vi "TLM.vi"(4 "Error In":errorcluster, 7 "Command":string) -> (0 "Error Out":errorcluster, 3 "Response":string)   [LabVIEW 2018]
uses:
  MOKO_LabViewLibrary/MokoLowLevel/MokoLowLovelControl/MLLC_Mode.ctl
  data/TLM.ctl
panel:
  in  "Utility name":string="TLM"
  in  "Error Code":i32=5475
  in  "Settings":T2
  in  "Mode":T3=enum."Check"
  # "TLM"
  # "Default Settings"
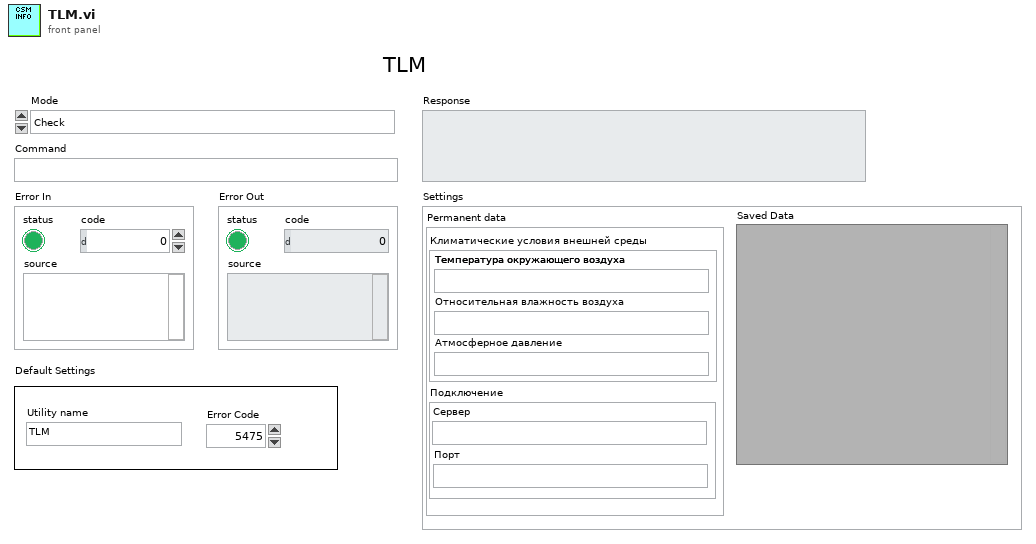
[diagram p1: front panel]
types:
  T1 = typedef "TLM.ctl" = cluster{"Климатические условия внешней среды":cluster{"Температура окружающего воздуха":string, "Относительная влажность воздуха":string, "Атмосферное давление":string}, "Подключение":cluster{"Сервер":string, "Порт":string}}
  T2 = cluster{"Saved Data":variant, "Permanent data":T1}
  T3 = typedef "MLLC_Mode.ctl" = enum16{"get", "set", "close", "Init", "Check"}
  T4 = typedef "MLLC_Error.ctl" = errorcluster
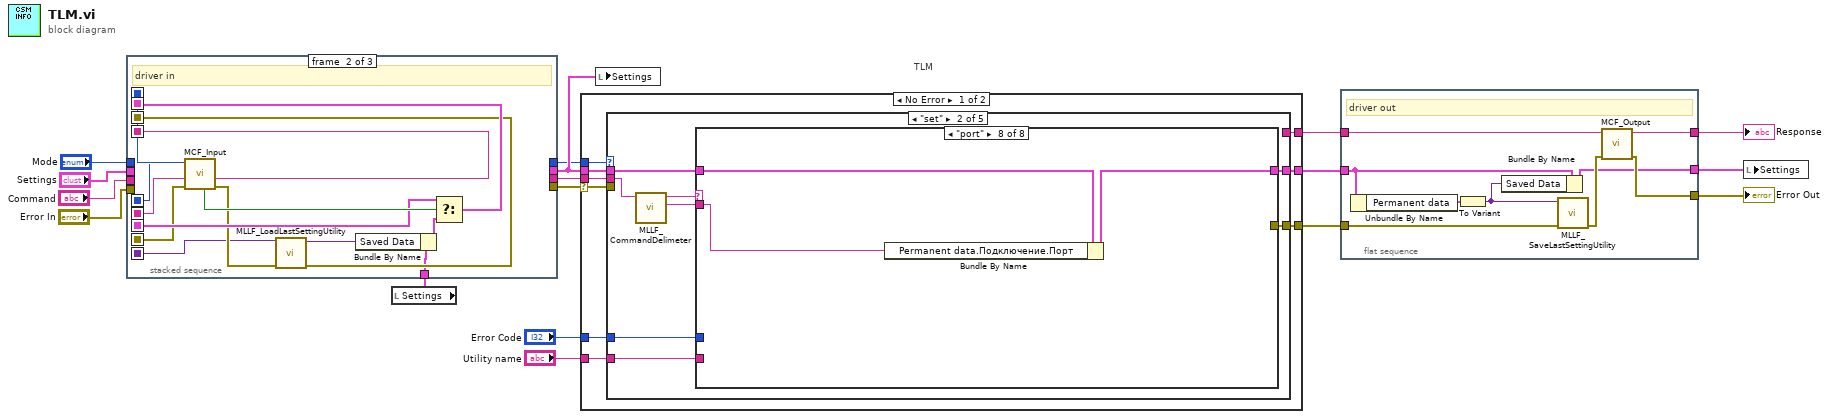
[diagram p0: block diagram]
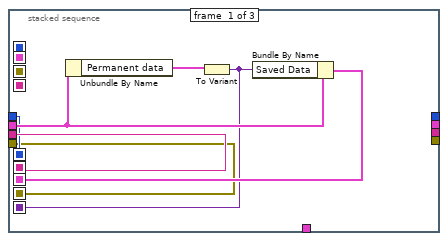
[diagram p2: hidden frame]
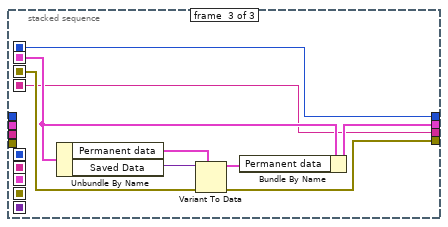
[diagram p3: hidden frame]
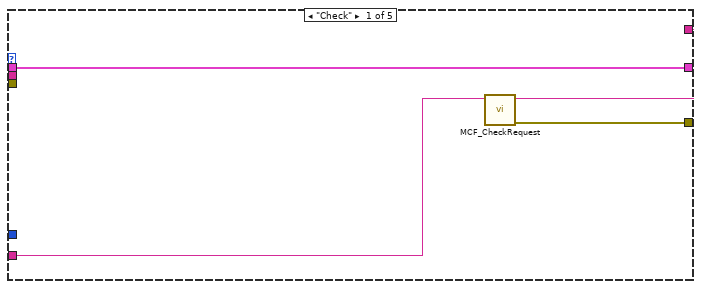
[diagram p4: hidden frame]
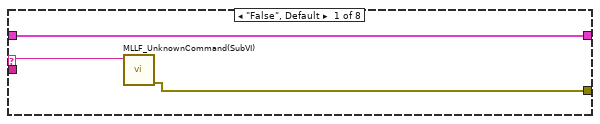
[diagram p5: hidden frame]
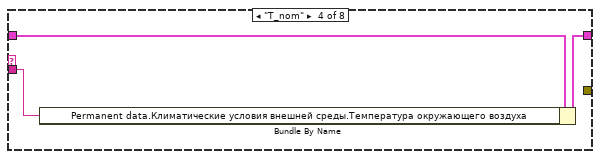
[diagram p8: hidden frame]
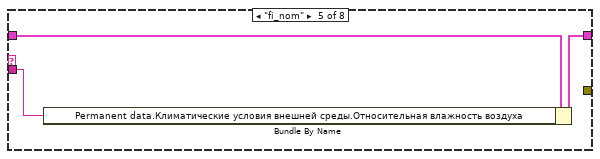
[diagram p9: hidden frame]
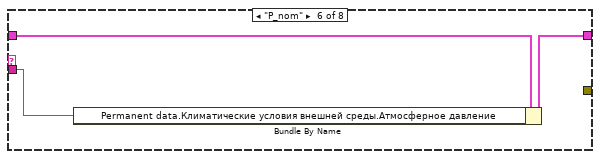
[diagram p10: hidden frame]
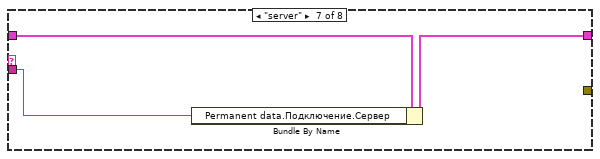
[diagram p11: hidden frame]
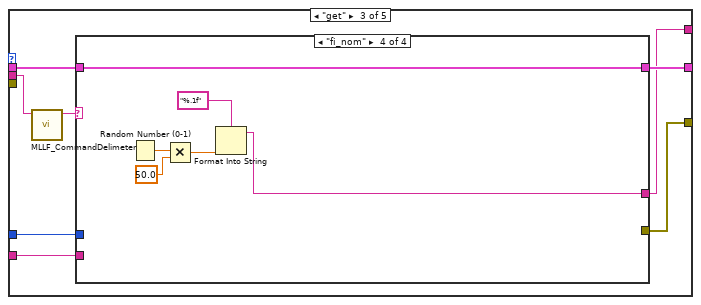
[diagram p12: hidden frame]
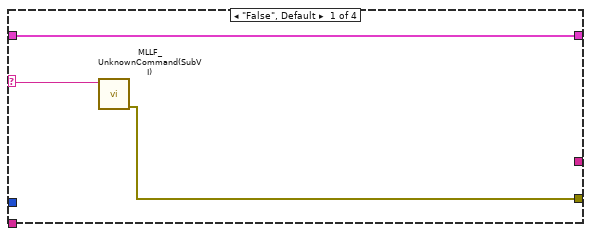
[diagram p13: hidden frame]
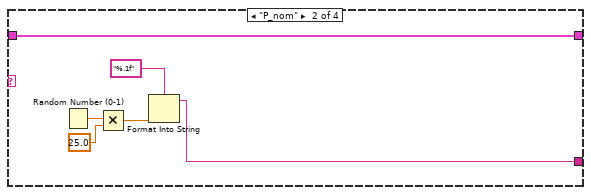
[diagram p14: hidden frame]
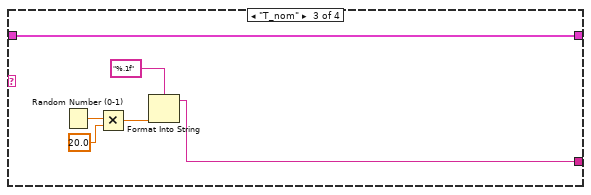
[diagram p15: hidden frame]
diagram:
  # "TLM"
  n1 = local read "Settings"() -> (w12:T2)
  n2 = stacked-sequence {
    seq-local: [w20 _ _] -> [_ w36 _]
    seq-local: [w19 _ _] -> [_ w37 _]
    seq-local: [w22 _ _] -> [_ w32 _]
    seq-local: [w18 _ _] -> [_ w31 _]
    seq-local: [w21 _ _] -> [_ w26 _]
    seq-local: [_ w27 _] -> [_ _ w43]
    seq-local: [_ w38 _] -> [_ _ w40]
    seq-local: [_ w35 _] -> [_ _ w39]
    seq-local: [_ w34 _] -> [_ _ w44]
    tunnel: "Command" -> [w20 _ _]
    tunnel: "Mode" -> [w19 _ _]
    tunnel: "Error In" -> [w18 _ _]
    tunnel: "Settings" -> [w23 _ _]
    tunnel: w12 -> [_ w25 _]
    tunnel: [_ _ w39] -> w8
    tunnel: [_ _ w42] -> w11
    tunnel: [_ _ w41] -> w10
    tunnel: [_ _ w40] -> w9
    frame #0 {
      n3 = Unbundle By Name(w23) -> ("Permanent data"=w24:T1)
      n4 = To Variant(anything=w24) -> (Variant=w21:variant)
      n5 = Bundle By Name(cluster=w23, "Saved Data"=w21) -> (w22:T2)
    }
    frame #1 {
      # "driver in"
      n6 = call "MCF_Input.vi"("error in (no error)"=w31, "Command"=w36, "Mode"=w37) -> ("error out"=w30:errorcluster, "Command out"=w35:string, "Mode out"=w38:T3, "Boolean"=w33:bool)  [unwired: 5 in]
      n7 = call "MLLF_LoadLastSettingUtility.vi"("Error In"=w30, "Save data in"=w26) -> ("Error Out"=w27:errorcluster, "Save data out"=w29:variant)  [unwired: 8 in]
      n8 = Bundle By Name(cluster=w25, "Saved Data"=w29) -> (w28:T2)
      n9 = Select(t=w32, s=w33, f=w28) -> (s? t:f=w34:T2)
    }
    frame #2 {
      n10 = Unbundle By Name(w44) -> ("Permanent data"=w45:T1, "Saved Data"=w47:variant)
      n11 = Variant To Data(error in=w43, type=w45, Variant=w47) -> (data=w46:T1, error out=w41:errorcluster)
      n12 = Bundle By Name(cluster=w44, "Permanent data"=w46) -> (w42:T2)
    }
  }
  n13 = case shown="No Error" w10 {
    selector: w10 -> [w52 w121]
    tunnel: [w54 w121] -> w16
    tunnel: w9 -> [w56 _]
    tunnel: [w55 _] -> w14
    tunnel: w8 -> [w53 _]
    tunnel: w11 -> [w49 w120]
    tunnel: "Error Code" -> [w51 _]
    tunnel: "Utility name" -> [w50 _]
    tunnel: [w48 w120] -> w15
    frame No Error {
      n14 = case shown="\"set\"" w56 {
        tunnel: [w58 _ w90 _ _] -> w55
        tunnel: [w57 w67 w89 _ _] -> w54
        tunnel: w53 -> [_ w68 w96 _ _]
        tunnel: w52 -> [_ _ _ _ _]
        tunnel: w51 -> [_ w66 w94 _ _]
        tunnel: w50 -> [w59 w63 w93 _ _]
        tunnel: w49 -> [w60 w65 w95 w118 w119]
        tunnel: [w60 w64 w92 w118 w119] -> w48
        frame "Check" {
          n15 = call "MCF_CheckRequest.vi"("Driver Name"=w59) -> ("Error Out"=w57:errorcluster, "Output String"=w58:string)  [unwired: 9 in]
        }
        frame "set" {
          n16 = call "MLLF_CommandDelimeter.vi"("command with param"=w68) -> ("param 1"=w61:string, "command"=w62:string)  [unwired: 7 in, 2 out]
          n17 = case shown="\"port\"" w62 {
            selector: w62 -> [w70 _ _ _ _ _ _ _]
            tunnel: w61 -> [_ _ _ w74 w77 w80 w83 w86]
            tunnel: [w69 _ _ _ _ _ _ _] -> w67
            tunnel: w66 -> [_ _ _ _ _ _ _ _]
            tunnel: w65 -> [w71 w72 w73 w76 w79 w82 w85 w88]
            tunnel: [w71 w72 w73 w75 w78 w81 w84 w87] -> w64
            tunnel: w63 -> [_ _ _ _ _ _ _ _]
            frame "False", Default {
              n18 = call "MLLF_UnknownCommand(SubVI).vi"("Unknown command"=w70) -> ("error out"=w69:errorcluster)  [unwired: 10 in]
            }
            frame "<----MAIN FUNCTIONS---->" {
            }
            frame "---------ADDITIONAL---------" {
            }
            frame "T_nom" {
              n19 = Bundle By Name(cluster=w76, "Permanent data.Климатические условия внешней среды.Температура окружающего воздуха"=w74) -> (w75:T2)
            }
            frame "fi_nom" {
              n20 = Bundle By Name(cluster=w79, "Permanent data.Климатические условия внешней среды.Относительная влажность воздуха"=w77) -> (w78:T2)
            }
            frame "P_nom" {
              n21 = Bundle By Name(cluster=w82, "Permanent data.Климатические условия внешней среды.Атмосферное давление"=w80) -> (w81:T2)
            }
            frame "server" {
              n22 = Bundle By Name(cluster=w85, "Permanent data.Подключение.Сервер"=w83) -> (w84:T2)
            }
            frame "port" {
              n23 = Bundle By Name(cluster=w88, "Permanent data.Подключение.Порт"=w86) -> (w87:T2)
            }
          }
        }
        frame "get" {
          n24 = call "MLLF_CommandDelimeter.vi"("command with param"=w96) -> ("command"=w91:string)  [unwired: 7 in, 3 out]
          n25 = case shown="\"fi_nom\"" w91 {
            selector: w91 -> [w98 _ _ _]
            tunnel: [w97 _ _ _] -> w89
            tunnel: w94 -> [_ _ _ _]
            tunnel: [w99 w105 w111 w117] -> w92
            tunnel: w95 -> [w99 w105 w111 w117]
            tunnel: w93 -> [_ _ _ _]
            tunnel: [_ w100 w106 w112] -> w90
            frame "False", Default {
              n26 = call "MLLF_UnknownCommand(SubVI).vi"("Unknown command"=w98) -> ("error out"=w97:errorcluster)  [unwired: 10 in]
            }
            frame "P_nom" {
              n27 = Random Number (0-1)() -> (number: 0 to 1=w104:dbl)
              n28 = Multiply(x=w104, y=25.0) -> (x*y=w102:dbl)
              n29 = Format Into String(format string="%.1f", w102) -> (resulting string=w100:string)  [unwired: 2 in, 1 out]
            }
            frame "T_nom" {
              n30 = Random Number (0-1)() -> (number: 0 to 1=w110:dbl)
              n31 = Multiply(x=w110, y=20.0) -> (x*y=w108:dbl)
              n32 = Format Into String(format string="%.1f", w108) -> (resulting string=w106:string)  [unwired: 2 in, 1 out]
            }
            frame "fi_nom" {
              n33 = Random Number (0-1)() -> (number: 0 to 1=w116:dbl)
              n34 = Multiply(x=w116, y=50.0) -> (x*y=w114:dbl)
              n35 = Format Into String(format string="%.1f", w114) -> (resulting string=w112:string)  [unwired: 2 in, 1 out]
            }
          }
        }
        frame "close" {
        }
        frame "Init" {
        }
      }
    }
    frame Error {
    }
  }
  n36 = local write "Settings"(w11) -> ()
  n37 = flat-sequence {
    tunnel: [w130] -> w6
    tunnel: [w129] -> w4
    tunnel: w14 -> [w128]
    tunnel: w16 -> [w127]
    tunnel: w15 -> [w123]
    tunnel: [w125] -> w13
    frame #0 {
      # "driver out"
      n38 = Unbundle By Name(w123) -> ("Permanent data"=w122:T1)
      n39 = To Variant(anything=w122) -> (Variant=w124:variant)
      n40 = Bundle By Name(cluster=w123, "Saved Data"=w124) -> (w125:T2)
      n41 = call "MLLF_SaveLastSettingUtility.vi"("error in"=w127, "Saved Data"=w124) -> ("error out"=w126:T4)  [unwired: 8 in, 1 out]
      n42 = call "MCF_Output.vi"("Error In"=w126, "Input"=w128) -> ("Error Out"=w129:errorcluster, "Output"=w130:string)  [unwired: 8 in]
    }
  }
  n43 = local write "Settings"(w13) -> ()
  "Response" <- w6
  "Error Out" <- w4
